vi "VectorNorm.vi"(8 "error in (no error)":errorcluster, 11 "Vector":dbl[](array[numeric])) -> (0 "error out":errorcluster, 3 "Norm":dbl)   [LabVIEW 2010]
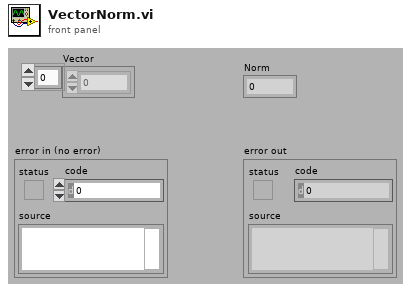
[diagram p1: front panel]
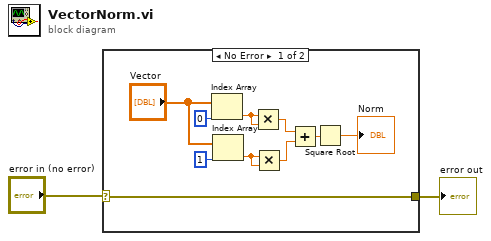
[diagram p0: block diagram]
diagram:
  n1 = case shown="No Error" "error in (no error)" {
    selector: "error in (no error)" -> [w3 w13]
    tunnel: [w3 w13] -> w1
    frame No Error {
      n2 = Index Array(array="Vector", index=0) -> (element=w7:dbl)
      n3 = Index Array(array="Vector", index=1) -> (element=w12:dbl)
      n4 = Multiply(x=w7, y=w7) -> (x*y=w10:dbl)
      n5 = Multiply(x=w12, y=w12) -> (x*y=w9:dbl)
      n6 = Add(x=w10, y=w9) -> (x+y=w11:dbl)
      n7 = Square Root(x=w11) -> (sqrt(x)=→"Norm":dbl)
    }
    frame Error {
    }
  }
  "error out" <- w1
